vi "Main.vi"() -> ()   [LabVIEW 2010]
panel:
  in  "stop":bool
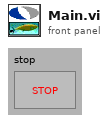
[diagram p1: front panel]
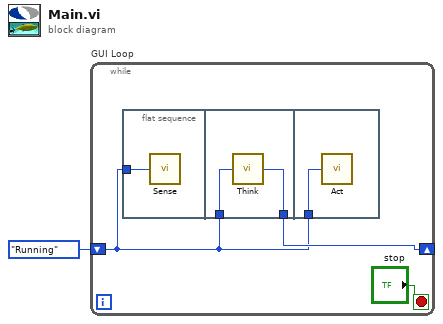
[diagram p0: block diagram]
diagram:
  n1 = while "GUI Loop" {
    shift-right: [w3] -> _
    shift-left: enum16{"Running", "Impact", "Spinning", "Clear"}."Running" -> [w2]
    stop <- "stop" stop-if-true
    n2 = flat-sequence {
      tunnel: w2 -> [w5]
      tunnel: [w7] -> w3
      tunnel: w2 -> [w6]
      tunnel: w2 -> [w8]
      frame #0 {
        n3 = call "Sense.vi"("Enum"=w5) -> ()
      }
      frame #1 {
        n4 = call "Think.vi"("Enum"=w6) -> ("Enum 2"=w7:enum16{"Running", "Impact", "Spinning", "Clear"})
      }
      frame #2 {
        n5 = call "Act.vi"("Enum"=w8) -> ()
      }
    }
  }
